vi "Set Content Type.vi"(8 "error in (no error)":errorcluster, 10 "Content Type (application/json)":string="application/json", 11 "Response in":refnum<class "Response.lvclass">) -> (0 "error out":errorcluster, 3 "Response out":refnum<class "Response.lvclass">)   [LabVIEW 2023, in "Response.lvclass"]
doc: "Set Response Content-Type. This is needed to help the client know how to interpret the body text."
uses:
  Response.lvclass
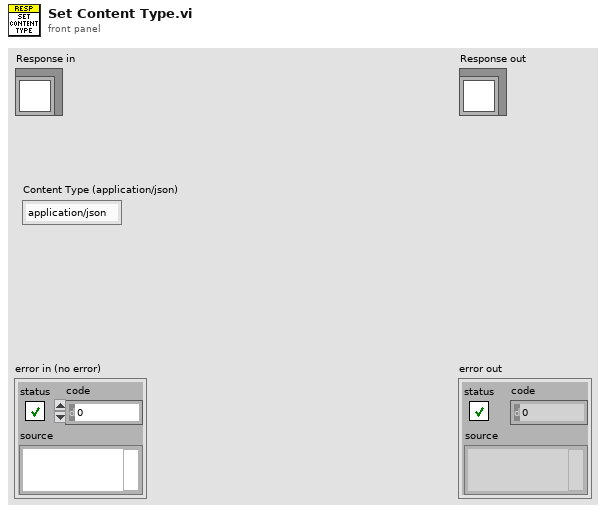
[diagram p1: front panel]
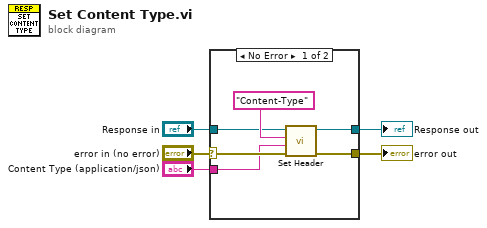
[diagram p0: block diagram]
diagram:
  n1 = case shown="No Error" "error in (no error)" {
    selector: "error in (no error)" -> [w7 w13]
    tunnel: [w11 w13] -> w4
    tunnel: [w10 w12] -> w2
    tunnel: "Response in" -> [w8 w12]
    tunnel: "Content Type (application/json)" -> [w6 _]
    frame No Error {
      n2 = call "Set Header.vi"("error in (no error)"=w7, "Value"=w6, "Header"="Content-Type", "Response in"=w8) -> ("error out"=w11:errorcluster, "Response out"=w10:refnum<class "Response.lvclass">)  [unwired: 5 in, 1 out]
    }
    frame Error {
    }
  }
  "error out" <- w4
  "Response out" <- w2
